vi "unflattenFromString.vi"(8 "error in (no error)":errorcluster, 10 "binary string":string, 11 "Worker Status in":refnum<class "Worker Status.lvclass">) -> (0 "error out":errorcluster, 3 "Worker Status out":refnum<class "Worker Status.lvclass">)   [LabVIEW 2017, in "Message Interface.lvlib" / "Worker Status.lvclass"]
uses:
  Worker Status.lvclass
  C:/Users/Public/Documents/wc/BuildFarm/src/LabVIEW/vi.lib/BenjaminR/Build Farm/Classes/Message Interface/Status/Status.lvclass
  Status/Status.lvclass/Status.ctl
  Status/Read Item Name.vi
  Status/Write Item Name.vi
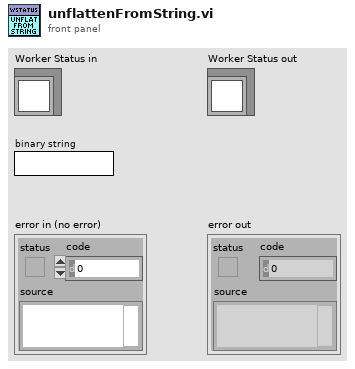
[diagram p1: front panel]
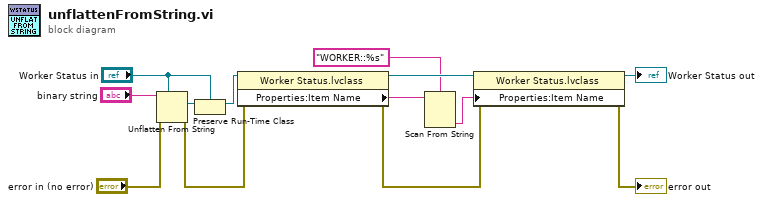
[diagram p0: block diagram]
diagram:
  n1 = Unflatten From String(type="Worker Status in", binary string="binary string", error in (no error)="error in (no error)") -> (value=w5:refnum<class "Worker Status.lvclass">, error out=w3:errorcluster)  [unwired: 2 in, 1 out]
  n2 = Preserve Run-Time Class(object in=w5, 2:"Worker Status in") -> (object out=w2:refnum<class "Worker Status.lvclass">)  [unwired: 1 in, 1 out]
  n3 = property class="Worker Status.lvclass"(reference=w2, error in=w3) -> (reference out=w13:refnum<class "Worker Status.lvclass">, error out=w10:errorcluster, "Properties:Item Name"=w9:string)
  n4 = Scan From String(format string="WORKER::%s" ("string"), input string=w9) -> (output 1=w7:string)  [unwired: 3 in, 3 out]
  n5 = property class="Worker Status.lvclass"(reference=w13, error in=w10, "Properties:Item Name"=w7) -> (reference out=→"Worker Status out":refnum<class "Worker Status.lvclass">, error out=→"error out":errorcluster)
